vi "Find Range Check Result by Multicolumn Listbox Value.vi"(3 "error in (no error)":errorcluster, 4 "reference":refnum<vi>, 5 "Range Check Results in":T2(array[cluster])=[{"name"="D:OUTTMP", "value"=17.051272696256788, "range state"=0}]) -> (0 "error out":errorcluster, 1 "Found?":bool, 2 "Range Check Result out":T1)   [LabVIEW 2013, in "ACNET Monitor.lvlib"]
uses:
  ACNET Monitor.lvlib
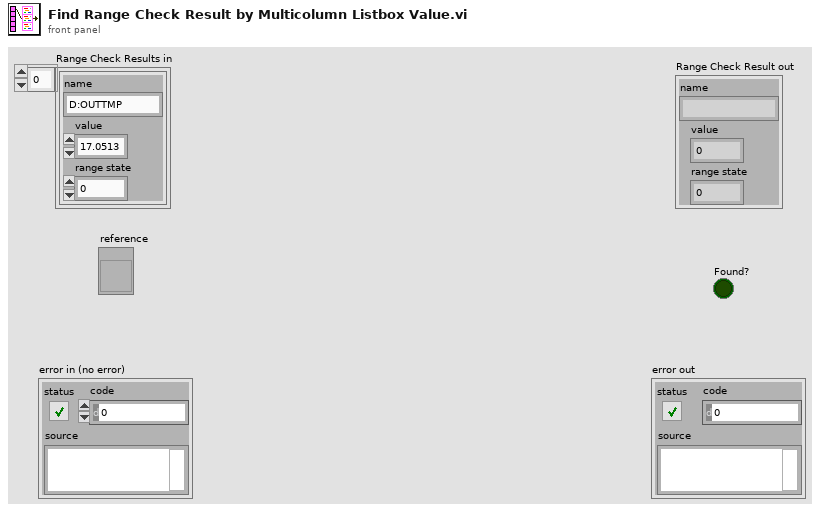
[diagram p1: front panel]
types:
  T1 = cluster{"name":string, "value":dbl, "range state":i8}
  T2 = cluster{"name":string, "value":dbl, "range state":i8}[]
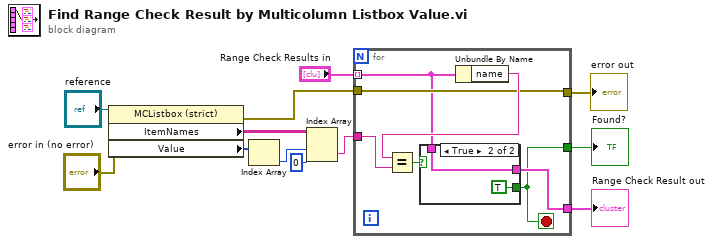
[diagram p0: block diagram]
diagram:
  n1 = property on="Property Node" class="MCListbox (strict)"(reference="reference", error in="error in (no error)") -> (error out=w5:errorcluster, "ItemNames"=w10:string[][], "Value"=w8:i32[])  [unwired: 1 out]
  n2 = Index Array(array=w8) -> (element=w11:i32)  [unwired: 1 in]
  n3 = Index Array(array=w10, index (row)=w11, index (col)=0 ("disabled index (col)")) -> (element=w12:string)
  n4 = for {
    tunnel: "Range Check Results in" -> [w13] mode=indexing
    tunnel: w5 -> [w14]
    tunnel: w12 -> [w18]
    tunnel: [w14] -> w6
    tunnel: [w16] -> w3
    tunnel: [w15] -> w2
    stop <- w15 stop-if-true
    n5 = Unbundle By Name(w13) -> ("name"=w19:string)
    n6 = Equal?(x=w19, y=w18) -> (x = y?=w17:bool)
    n7 = case shown="True" w17 {
      tunnel: [_ TRUE] -> w15
      tunnel: w13 -> [_ w20]
      tunnel: [_ w20] -> w16
      frame False {
      }
      frame True {
      }
    }
  }
  "error out" <- w6
  "Range Check Result out" <- w3
  "Found?" <- w2
